vi "二维数组排序(str).vi"(1 "数组输入":string[][](array[string])) -> (0 "数组输出":string[][](array[string]))   [LabVIEW 2014, in "数组操作.lvlib"]
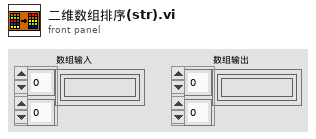
[diagram p1: front panel]
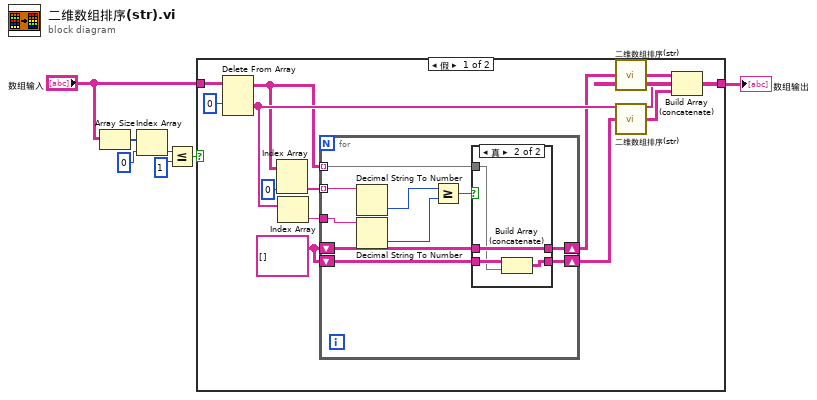
[diagram p0: block diagram]
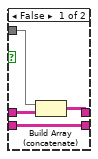
[diagram p2: hidden frame]
diagram:
  n1 = Array Size(array="数组输入") -> (size(s)=w3:i32[])
  n2 = Index Array(array=w3, index=0 ("y")) -> (element=w4:i32)
  n3 = Less Or Equal?(x=w4, y=1) -> (x <= y?=w7:bool)
  n4 = case shown="假" w7 {
    tunnel: "数组输入" -> [w19 w39]
    tunnel: [w12 w39] -> w5
    frame False {
      w17 = string[][] [] ("数组")
      n5 = Delete From Array(array=w19, index (row)=0 ("索引")) -> (deleted portion=w20:string[], array with subset deleted=w9:string[][])  [unwired: 2 in]
      n6 = Index Array(array=w9, index (col)=0 ("禁用的索引 (列)")) -> (element=w11:string[])  [unwired: 1 in]
      n7 = Index Array(array=w20) -> (element=w8:string)  [unwired: 1 in]
      n8 = for {
        shift-right: [w27] -> w14
        shift-left: w17 -> [w26]
        shift-right: [w28] -> w13
        shift-left: w17 -> [w29]
        tunnel: w11 -> [w24] mode=indexing
        tunnel: w9 -> [w25] mode=indexing
        tunnel: w8 -> [w23]
        n9 = Decimal String To Number(string=w24) -> (number=w22:i32)  [unwired: 2 in, 1 out]
        n10 = Decimal String To Number(string=w23) -> (number=w21:i32)  [unwired: 2 in, 1 out]
        n11 = Greater Or Equal?(x=w22, y=w21) -> (x >= y?=w30:bool)
        n12 = case shown="真" w30 {
          tunnel: w29 -> [w32 w38]
          tunnel: [w32 w37] -> w28
          tunnel: [w34 w36] -> w27
          tunnel: w26 -> [w33 w36]
          tunnel: w25 -> [w31 w35]
          frame False {
            n13 = Build Array (concatenate)(w31, w33) -> (w34:string[][])
          }
          frame True {
            n14 = Build Array (concatenate)(w38, w35) -> (w37:string[][])
          }
        }
      }
      n15 = call "二维数组排序(str).vi"("数组输入"=w14) -> ("数组输出"=w16:string[][])
      n16 = call "二维数组排序(str).vi"("数组输入"=w13) -> ("数组输出"=w15:string[][])
      n17 = Build Array (concatenate)(w16, w20, w15) -> (w12:string[][])
    }
    frame True {
    }
  }
  "数组输出" <- w5
